vi "gfitsio-close-file.vi"(8 "error in (no error)":errorcluster, 11 "gfits refnum":T1) -> (0 "error out":errorcluster, 3 "Path":path)   [LabVIEW 2011, in "gfitsio.lvlib"]
doc: "Closes an open file specified by <B>gfits refnum</B>. Error I/O operates uniquely in this function, which closes the file regardless of whether an error occurred in a preceding operation."
uses:
  gfitsio.lvlib
  gfitsio-refnum.ctl
  gfitsio.dll
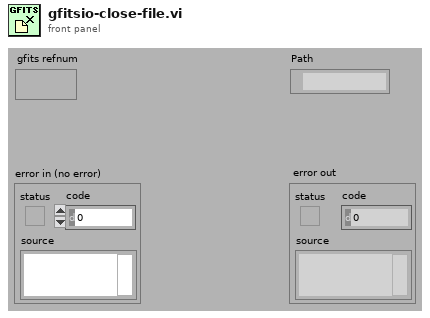
[diagram p1: front panel]
types:
  T1 = typedef "gfitsio.lvlib/gfitsio-refnum.ctl" = refnum<k1>
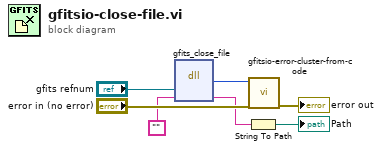
[diagram p0: block diagram]
diagram:
  n1 = dll-call lib="C:/jul 1 BonOmm 2.0/SubVIs/gfitsio/gfitsio.dll" fn="gfits_close_file"("gfits refnum"="gfits refnum", "path"="") -> (w7:i32, "path"=w3:string)  [unwired: 4 in, 2 out]
  n2 = String To Path(string=w3) -> (path=→"Path":path)
  n3 = call "gfitsio-error-cluster-from-code.vi"("error in (no error)"="error in (no error)", "error code"=w7) -> ("error out"=→"error out":errorcluster)  [unwired: 9 in]
